vi "FL Plot Variable.vi"(5 "variable index":i32, 7 "input/output":enum16{"Input", "Output"}(ring), 8 "error in (no error)":errorcluster, 10 "graph refnum":refnum<vi>, 11 "fuzzy system in":T1 {"user MF interpolating polynomials"."coa_x(y) coeff" format="%.4g"; "user MF interpolating polynomials"."Area(y) coeff" format="%.4g"; "user MF interpolating polynomials"."X(y) coeff" format="%.4g"; "user MF interpolating polynomials"."Y(x) coeff" format="%.4g"; "user MF interpolating polynomials"."Y" format="%.4g"; "user MF interpolating polynomials"."X" format="%.4g"; "defuzzification method" items=["Center of Area", "Modified Center of Area", "Center of Sums", "Center of Maximum", "Mean of Maximum"]; "rules"."consequents"."Var Index" min=0; "rules"."consequents"."Cond" items=["=", "!="]; "rules"."consequents"."MF Index" min=0; "rules"."antecedents"."Var Index" min=0; "rules"."antecedents"."Cond" items=["=", "!="]; "rules"."antecedents"."MF Index" min=0; "rules"."consequent implication" items=["Minimum", "Product"]; "rules"."antecedent connective" items=["AND (Minimum)", "AND (Product)", "OR (Maximum)", "OR (Probabilistic)"]; "output variables"."MFs"."shape" items=["Triangle", "Trapezoid", "Singleton", "Sigmoid", "Gaussian", "User-Defined"]; "input variables"."MFs"."shape" items=["Triangle", "Trapezoid", "Singleton", "Sigmoid", "Gaussian", "User-Defined"]}) -> (0 "error out":errorcluster, 2 "plot data (XY)":cluster{cluster{"Xi":dbl, "Yi":dbl}[]}[](array[cluster]), 3 "fuzzy system out":T1 {"user MF interpolating polynomials"."coa_x(y) coeff" format="%.4g"; "user MF interpolating polynomials"."Area(y) coeff" format="%.4g"; "user MF interpolating polynomials"."X(y) coeff" format="%.4g"; "user MF interpolating polynomials"."Y(x) coeff" format="%.4g"; "user MF interpolating polynomials"."Y" format="%.4g"; "user MF interpolating polynomials"."X" format="%.4g"; "defuzzification method" items=["Center of Area", "Modified Center of Area", "Center of Sums", "Center of Maximum", "Mean of Maximum"]; "rules"."consequents"."Var Index" min=0; "rules"."consequents"."Cond" items=["=", "!="]; "rules"."consequents"."MF Index" min=0; "rules"."antecedents"."Var Index" min=0; "rules"."antecedents"."Cond" items=["=", "!="]; "rules"."antecedents"."MF Index" min=0; "rules"."consequent implication" items=["Minimum", "Product"]; "rules"."antecedent connective" items=["AND (Minimum)", "AND (Product)", "OR (Maximum)", "OR (Probabilistic)"]; "output variables"."MFs"."shape" items=["Triangle", "Trapezoid", "Singleton", "Sigmoid", "Gaussian", "User-Defined"]; "input variables"."MFs"."shape" items=["Triangle", "Trapezoid", "Singleton", "Sigmoid", "Gaussian", "User-Defined"]})   [LabVIEW 2013, in "NI_Fuzzy_Logic_API.lvlib"]
uses:
  <vilib>/addons/Fuzzy Logic/NI_Fuzzy_Logic_API.lvlib
  <vilib>/addons/Fuzzy Logic/TypeDefs/FL System.ctl
  <vilib>/addons/Fuzzy Logic/TypeDefs/FL Variable.ctl
  <vilib>/addons/Fuzzy Logic/TypeDefs/FL Membership Function.ctl
  <vilib>/addons/Fuzzy Logic/TypeDefs/FL Membership Function Shape.ctl
  <vilib>/addons/Fuzzy Logic/TypeDefs/FL Rule.ctl
  <vilib>/addons/Fuzzy Logic/TypeDefs/FL Antecedent.ctl
  <vilib>/addons/Fuzzy Logic/TypeDefs/FL Modifier.ctl
  <vilib>/addons/Fuzzy Logic/TypeDefs/FL Antecedent Connective.ctl
  <vilib>/addons/Fuzzy Logic/TypeDefs/FL Consequent.ctl
  <vilib>/addons/Fuzzy Logic/TypeDefs/FL Consequent Implication.ctl
  <vilib>/addons/Fuzzy Logic/TypeDefs/FL Defuzzification.ctl
  <vilib>/addons/Fuzzy Logic/TypeDefs/FL Interpolating polynomials.ctl
  <vilib>/Analysis/1siggen.llb/Ramp Pattern by Samples.vi
  <vilib>/Analysis/NI_AALBase.lvlib
panel:
  out "graph error":errorcluster
  # "IF"
  # "THEN"
  # "IF"
  # "THEN"
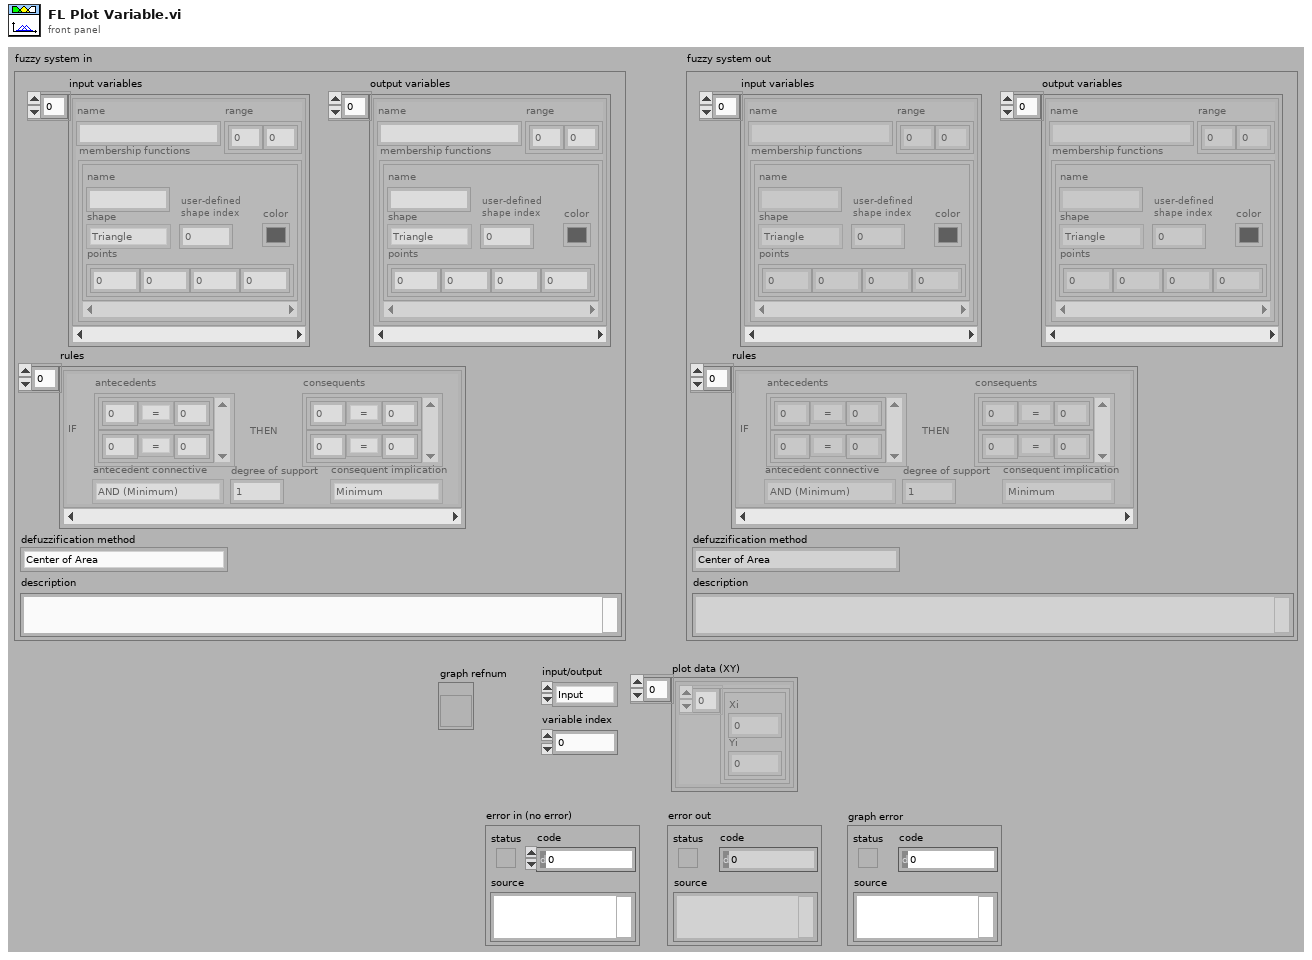
[diagram p1: front panel]
types:
  T1 = typedef "NI_Fuzzy_Logic_API.lvlib/FL System.ctl" = cluster{"input variables":T2[], "output variables":T2[], "rules":T5[], "defuzzification method":T11, "description":string, "user MF interpolating polynomials":T12[]}
  T2 = typedef "NI_Fuzzy_Logic_API.lvlib/FL Variable.ctl" = cluster{"name":string, "range":dbl[], "MFs":T3[]}
  T3 = typedef "NI_Fuzzy_Logic_API.lvlib/FL Membership Function.ctl" = cluster{"name":string, "shape":T4, "points":dbl[], "color":u32, "user-defined shape index":i32}
  T4 = typedef "NI_Fuzzy_Logic_API.lvlib/FL Membership Function Shape.ctl" = u16
  T5 = typedef "NI_Fuzzy_Logic_API.lvlib/FL Rule.ctl" = cluster{"antecedents":T6[], "antecedent connective":T8, "consequents":T9[], "consequent implication":T10, "degree of support":dbl}
  T6 = typedef "NI_Fuzzy_Logic_API.lvlib/FL Antecedent.ctl" = cluster{"Var Index":i32, "MF Index":i32, "Cond":T7}
  T7 = typedef "NI_Fuzzy_Logic_API.lvlib/FL Modifier.ctl" = u16
  T8 = typedef "NI_Fuzzy_Logic_API.lvlib/FL Antecedent Connective.ctl" = u16
  T9 = typedef "NI_Fuzzy_Logic_API.lvlib/FL Consequent.ctl" = cluster{"Var Index":i32, "MF Index":i32, "Cond":T7}
  T10 = typedef "NI_Fuzzy_Logic_API.lvlib/FL Consequent Implication.ctl" = u16
  T11 = typedef "NI_Fuzzy_Logic_API.lvlib/FL Defuzzification.ctl" = u16
  T12 = typedef "NI_Fuzzy_Logic_API.lvlib/FL Interpolating polynomials.ctl" = cluster{"X":dbl[], "Y":dbl[], "Y(x) coeff":dbl[][], "X(y) coeff":dbl[][], "Area(y) coeff":dbl[][], "coa_x(y) coeff":dbl[][]}
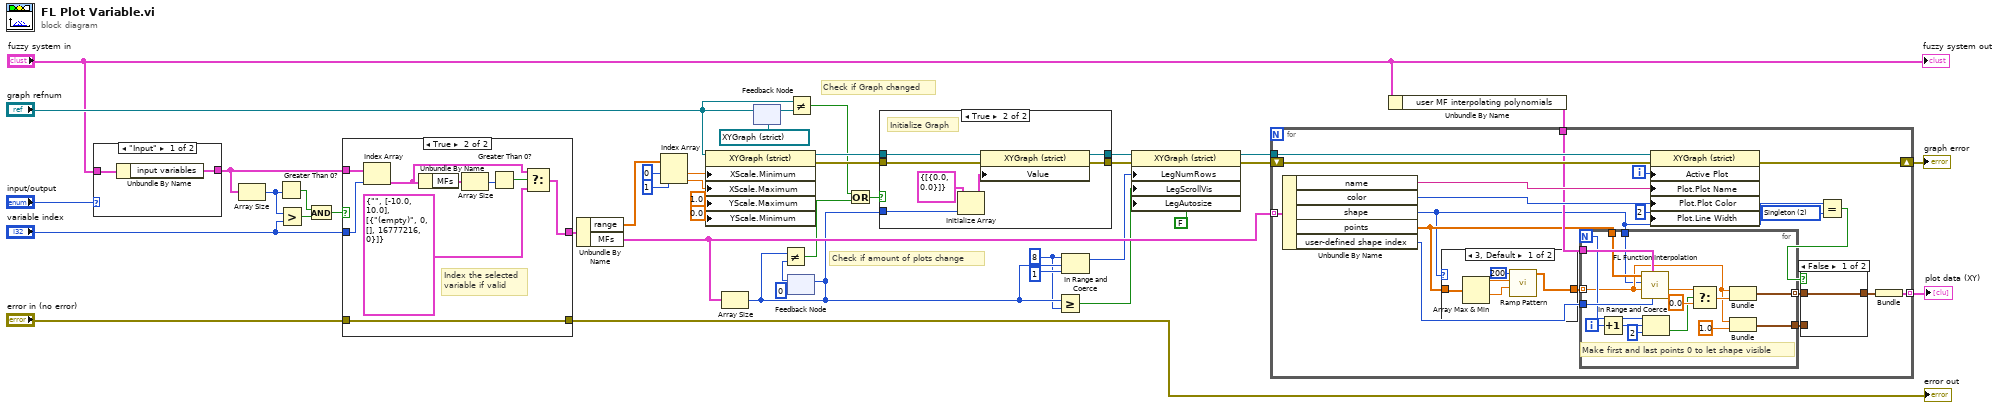
[diagram p0: block diagram]
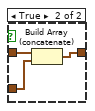
[diagram p2: hidden frame]
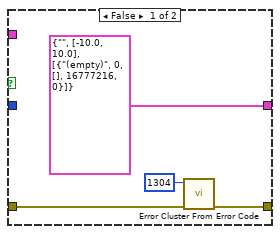
[diagram p4: hidden frame]
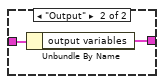
[diagram p5: hidden frame]
diagram:
  w8 = 8 ("upper limit")
  # "Check if Graph changed"
  # "Check if amount of plots change"
  n1 = case shown="\"Input\"" "input/output" {
    tunnel: "fuzzy system in" -> [w44 w46]
    tunnel: [w43 w45] -> w29
    frame "Input" {
      n2 = Unbundle By Name(w44) -> ("input variables"=w43:T2[])
    }
    frame "Output" {
      n3 = Unbundle By Name(w46) -> ("output variables"=w45:T2[])
    }
  }
  n4 = Array Size(array=w29) -> (size(s)=w32:i32)
  n5 = Greater Than 0?(x=w32) -> (x > 0?=w31:bool)
  n6 = Greater?(x=w32, y="variable index") -> (0:w33:bool)
  n7 = And(x=w31, y=w33) -> (x .and. y?=w30:bool)
  n8 = case shown="True" w30 {
    tunnel: [T2 {"name"="", "range"=[-10.0, 10.0], "MFs"=[{"name"="(empty)", "shape"=0, "points"=[], "color"=16777216, "user-defined shape index"=0}]} ("Variable") w52] -> w26
    tunnel: w29 -> [_ w59]
    tunnel: "variable index" -> [_ w58]
    tunnel: [w48 w57] -> w18
    tunnel: "error in (no error)" -> [w49 w57]
    frame False {
      n9 = call <vilib>:"Error Cluster From Error Code.vi"("error in (no error)"=w49, "error code (0)"=1304) -> ("error out"=w48:errorcluster)  [unwired: 1 in, 6 out]
    }
    frame True {
      # "Index the selected\nvariable if valid"
      n10 = Index Array(array=w59, index=w58) -> (element=w53:T2)
      n11 = Unbundle By Name(w53) -> ("MFs"=w55:T3[])
      n12 = Array Size(array=w55) -> (size(s)=w56:i32)
      n13 = Greater Than 0?(x=w56) -> (x > 0?=w54:bool)
      n14 = Select(t=w53, s=w54, f=T2 {"name"="", "range"=[-10.0, 10.0], "MFs"=[{"name"="(empty)", "shape"=0, "points"=[], "color"=16777216, "user-defined shape index"=0}]} ("Variable")) -> (s? t:f=w52:T2)
    }
  }
  "error out" <- w18
  n15 = Unbundle By Name(w26) -> ("range"=w5:dbl[], "MFs"=w38:T3[])
  n16 = Index Array(array=w5, index #1=0 ("index"), index #2=1 ("index")) -> (element #1=w2:dbl, element #2=w1:dbl)
  n17 = property on="Property Node" class="XYGraph (strict)"(reference="graph refnum", "XScale.Minimum"=w2, "XScale.Maximum"=w1, "YScale.Maximum"=1.0 ("Y Scale.Range:Maximum"), "YScale.Minimum"=0.0 ("Y Scale.Range:Minimum")) -> (reference out=w41:refnum<vi>, error out=w25:errorcluster)  [unwired: 1 in]
  n18 = Array Size(array=w38) -> (size(s)=w21:i32)
  n19 = feedback-in #1("graph refnum") -> ()
  n20 = feedback #1(refnum<vi> refnum ("Graph Refnum")) -> (w15:refnum<vi>)
  n21 = feedback-in #2(w21) -> ()
  n22 = feedback #2(0) -> (w22:i32)
  n23 = Not Equal?(x=w21, y=w22) -> (x != y?=w20:bool)
  n24 = Not Equal?(x="graph refnum", y=w15) -> (x != y?=w13:bool)
  n25 = Or(x=w13, y=w20) -> (x .or. y?=w19:bool)
  n26 = case shown="True" w19 {
    tunnel: w41 -> [w61 w68]
    tunnel: [w61 w63] -> w39
    tunnel: w25 -> [w60 w67]
    tunnel: [w60 w62] -> w24
    tunnel: w21 -> [_ w64]
    frame False {
    }
    frame True {
      # "Initialize Graph"
      n27 = Initialize Array(cluster{"Function Graph":cluster{dbl, dbl}[]} {"Function Graph"=[{0.0, 0.0}]}, w64) -> (w65:cluster{"Function Graph":cluster{dbl, dbl}[]}[])
      n28 = property on="Property Node" class="XYGraph (strict)"(reference=w68, error in=w67, "Value"=w65) -> (reference out=w63:refnum<vi>, error out=w62:errorcluster)
    }
  }
  n29 = Greater Or Equal?(x=w21, y=w8) -> (x >= y?=w35:bool)
  n30 = In Range and Coerce(upper limit=w8, x=w21, lower limit=1) -> (coerced(x)=w37:i32)  [unwired: 1 out]
  n31 = property on="Property Node" class="XYGraph (strict)"(reference=w39, error in=w24, "LegNumRows"=w37, "LegScrollVis"=w35, "LegAutosize"=FALSE ("Legend:Autosize")) -> (reference out=w40:refnum<vi>, error out=w23:errorcluster)
  n32 = Unbundle By Name("fuzzy system in") -> ("user MF interpolating polynomials"=w7:T12[])
  n33 = for {
    tunnel: w38 -> [w85] mode=indexing
    tunnel: w40 -> [w83]
    tunnel: [w82] -> w42 mode=indexing
    shift-right: [w80] -> w17
    shift-left: w23 -> [w81]
    tunnel: w7 -> [w79]
    i -> [w84]
    w74 = T4 2 items=["Triangle", "Trapezoid", "Singleton", "Sigmoid", "Gaussian", "User-Defined"] ("y")
    n34 = Unbundle By Name(w85) -> ("name"=w86:string, "color"=w87:u32, "shape"=w73:T4, "points"=w77:dbl[], "user-defined shape index"=w75:i32)
    n35 = case shown="3, Default" w73 {
      tunnel: [w92 w97] -> w78
      tunnel: w77 -> [w94 w97]
      frame 3, Default {
        n36 = Array Max & Min(array=w94) -> (max value=w96:dbl, min value=w95:dbl)  [unwired: 2 out]
        n37 = call-poly <vilib>:"Ramp Pattern.vi"("start"=w95, "end"=w96, "samples"=200) -> ("Ramp Pattern"=w92:dbl[])  [unwired: 7 in, 1 out]
      }
      frame 0..2 {
      }
    }
    n38 = for {
      N -> [w106]
      tunnel: w79 -> [w113]
      tunnel: w78 -> [w102] mode=indexing
      tunnel: [w99] -> w71 mode=indexing
      tunnel: w73 -> [w100]
      tunnel: w77 -> [w112]
      tunnel: w75 -> [w111]
      tunnel: [w98] -> w69
      i -> [w105]
      # "Make first and last points 0 to let shape visible"
      n39 = Increment(x=w105) -> (x+1=w104:i32)
      n40 = call <vilib>:"FL Function Interpolation.vi"("user-defined \nshape index"=w111, "user MF interpolating polynomials"=w113, "Input Data"=w102, "shape"=w100, "Points"=w112) -> ("Membership"=w108:dbl)  [unwired: 1 in, 5 out]
      n41 = In Range and Coerce(upper limit=w106, x=w104, lower limit=2) -> (In Range?=w103:bool)  [unwired: 1 out]
      n42 = Select(t=w108, s=w103, f=0.0) -> (s? t:f=w109:dbl)
      n43 = Bundle("Numeric"=w102, "f"=w109) -> (w99:cluster{"Numeric":dbl, "f":dbl})  [unwired: 1 out]
      n44 = Bundle("Numeric"=w102, "f"=1.0) -> (w98:cluster{"Numeric":dbl, "f":dbl})  [unwired: 1 out]
    }
    n45 = property on="Property Node" class="XYGraph (strict)"(reference=w83, error in=w81, "Active Plot"=w84, "Plot.Plot Name"=w86, "Plot.Plot Color"=w87, "Plot.Line Width"=u8 2) -> (error out=w80:errorcluster)  [unwired: 1 out]
    n46 = Equal?(x=w73, y=w74) -> (x = y?=w72:bool)
    n47 = case shown="False" w72 {
      tunnel: w71 -> [w88 w91]
      tunnel: [w88 w89] -> w70
      tunnel: w69 -> [_ w90]
      frame False {
      }
      frame True {
        n48 = Build Array (concatenate)(w91, w90) -> (w89:cluster{"Numeric":dbl, "f":dbl}[])
      }
    }
    n49 = Bundle(w70) -> (w82:cluster{cluster{"Numeric":dbl, "f":dbl}[]})  [unwired: 1 in]
  }
  "plot data (XY)" <- w42
  "graph error" <- w17
  "fuzzy system out" <- "fuzzy system in"
